vi "Practica3.vi"() -> ()   [LabVIEW 2014]
uses:
  <vilib>/Analysis/7linalg.llb/Solve Linear Equations (single right hand).vi
  <vilib>/Analysis/baseanly.llb/Solve Linear Equations By Cholesky.vi
  <vilib>/Analysis/baseanly.llb/Real Matrix to Compact Array.vi
  <vilib>/Analysis/baseanly.llb/Real Compact Tri-Matrix Linear Eqs.vi
  <vilib>/Analysis/7linalg.llb/Solve Linear Eqs (General).vi
  <vilib>/Analysis/7linalg.llb/Solve Linear Eqs (Gen, single right hand).vi
  <vilib>/Analysis/NI_AALPro.lvlib
panel:
  in  "stop":bool
  in  "OK Button":bool
  out "element 3":dbl
  out "element 2":dbl
  out "element":dbl
  in  "T1":dbl format="%#_13g"
  in  "T2":dbl format="%#_13g"
  in  "T3":dbl format="%#_13g"
  in  "R en T3":dbl format="%#_13g"
  in  "R en T2":dbl format="%#_13g"
  in  "R en T1":dbl format="%#_13g"
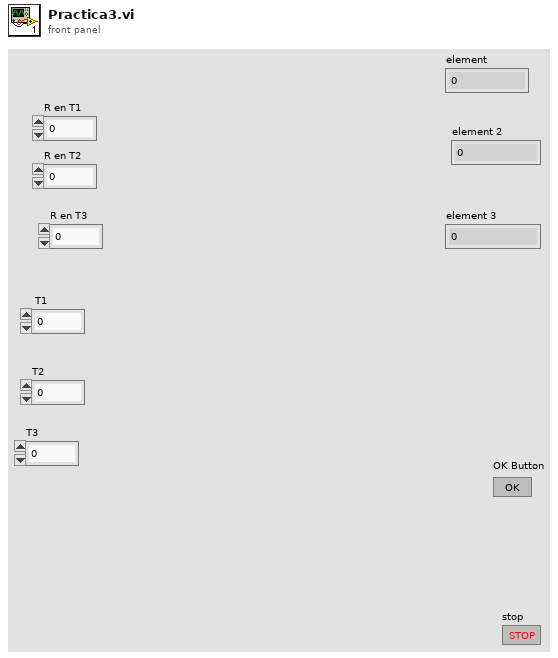
[diagram p1: front panel]
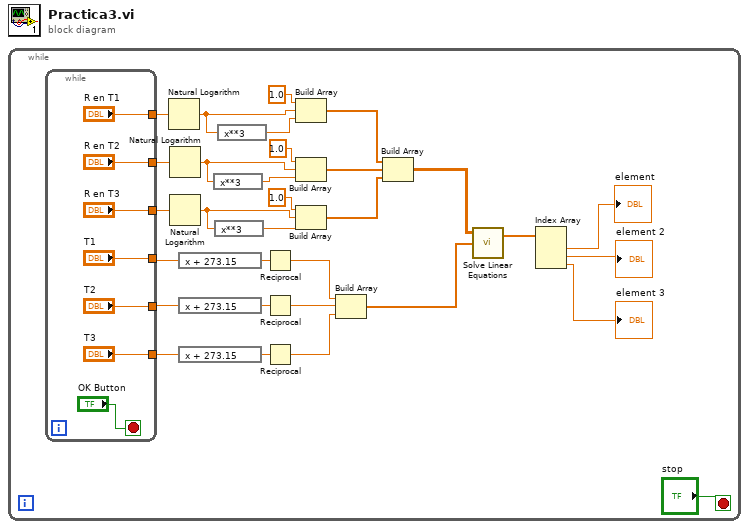
[diagram p0: block diagram]
diagram:
  n1 = while {
    stop <- "stop" stop-if-true
    n2 = while {
      tunnel: ["R en T1"] -> w22
      tunnel: ["R en T2"] -> w21
      tunnel: ["R en T3"] -> w20
      tunnel: ["T1"] -> w31
      tunnel: ["T2"] -> w30
      tunnel: ["T3"] -> w29
      stop <- "OK Button" stop-if-true
    }
    n3 = Natural Logarithm(1:w22) -> (0:w12:dbl)
    n4 = Natural Logarithm(1:w21) -> (0:w15:dbl)
    n5 = Natural Logarithm(1:w20) -> (0:w18:dbl)
    n6 = expression code="x + 273.15"(w31) -> (w28:dbl)
    n7 = expression code="x + 273.15"(w30) -> (w27:dbl)
    n8 = expression code="x + 273.15"(w29) -> (w26:dbl)
    n9 = expression code="x**3"(w15) -> (w16:dbl)
    n10 = expression code="x**3"(w18) -> (w19:dbl)
    n11 = expression code="x**3"(w12) -> (w13:dbl)
    n12 = Reciprocal(x=w28) -> (1/x=w25:dbl)
    n13 = Reciprocal(x=w27) -> (1/x=w23:dbl)
    n14 = Reciprocal(x=w26) -> (1/x=w24:dbl)
    n15 = Build Array(1.0 ("element"), w12, w13) -> (w10:dbl[])
    n16 = Build Array(1.0 ("element"), w15, w16) -> (w9:dbl[])
    n17 = Build Array(1.0 ("element"), w18, w19) -> (w8:dbl[])
    n18 = Build Array(w25, w23, w24) -> (w6:dbl[])
    n19 = Build Array(w10, w9, w8) -> (w7:dbl[][])
    n20 = call-poly <vilib>:"Solve Linear Equations.vi"("Known Vector"=w6, "Input Matrix"=w7) -> ("Solution Vector"=w5:dbl[])  [unwired: 1 in, 1 out]
    n21 = Index Array(array=w5) -> (element #1=→"element":dbl, element #2=→"element 2":dbl, element #3=→"element 3":dbl)  [unwired: 3 in]
  }
